vi "Decode Points Referee.vi"(7 "Boolean":bool=TRUE, 8 "error in":errorcluster, 9 "array":u8[](array[numeric]), 10 "Key":i32=5) -> (0 "error out":errorcluster, 1 "array w/ subset deleted out":u8[](array[numeric]), 3 "Point":cluster{"x":sgl, "y":sgl})   [LabVIEW 2023]
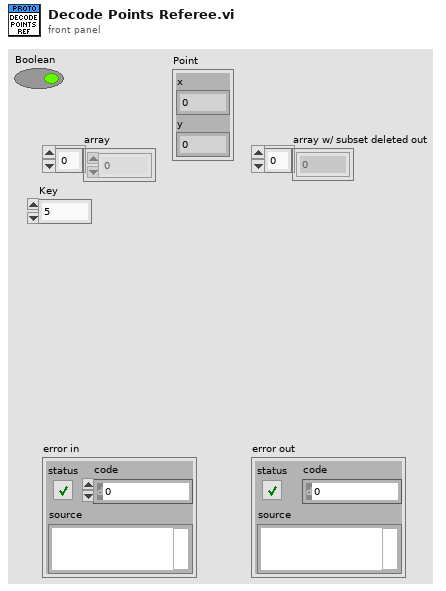
[diagram p1: front panel]
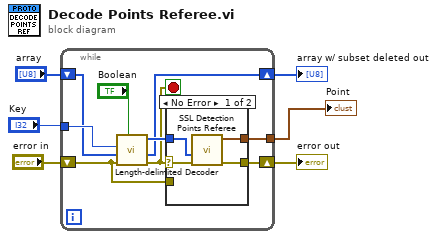
[diagram p0: block diagram]
diagram:
  n1 = while {
    shift-right: [w13] -> w4
    shift-left: "array" -> [w9]
    shift-right: [w15] -> w6
    shift-left: "error in" -> [w12]
    tunnel: "Key" -> [w10]
    tunnel: [w8] -> w1
    stop <- w11 stop-if-true
    n2 = call "Length-delimited Decoder.vi"("Optional"="Boolean", "error in (no error)"=w12, "Array"=w9, "Key"=w10) -> ("error out"=w11:errorcluster, "array w/ subset deleted"=w13:u8[], "Length-delimited"=w14:u8[])  [unwired: 4 in, 1 out]
    n3 = case shown="No Error" w11 {
      selector: w11 -> [w18 _]
      tunnel: [w19 w20] -> w15
      tunnel: w14 -> [w17 _]
      tunnel: w12 -> [_ w20]
      tunnel: [w16 _] -> w8
      frame No Error {
        n4 = call "SSL Detection Points Referee.vi"("error in"=w18, "Array"=w17) -> ("error out"=w19:errorcluster, "Point"=w16:cluster{"x":sgl, "y":sgl})  [unwired: 7 in, 1 out]
      }
      frame Error {
      }
    }
  }
  "error out" <- w6
  "array w/ subset deleted out" <- w4
  "Point" <- w1
